vi "DriveHalt.vi"(1 "Parameter String":string, 2 "Reinit":bool) -> (0 "Increment":bool)   [LabVIEW 2019]
uses:
  dsinstructions.vi
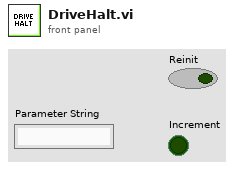
[diagram p1: front panel]
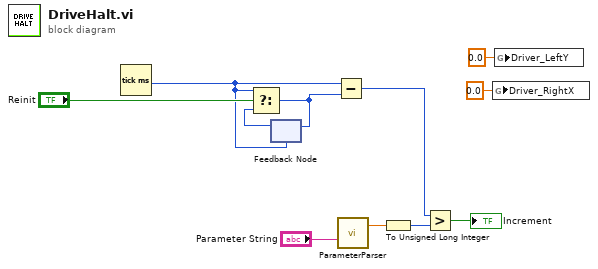
[diagram p0: block diagram]
diagram:
  n1 = Tick Count (ms)() -> (millisecond timer value=w4:u32)
  n2 = feedback #1(w4) -> (w10:u32)
  n3 = Select(t=w4, s="Reinit", f=w10) -> (s? t:f=w8:u32)
  n4 = feedback-in #1(w8) -> ()
  n5 = Subtract(x=w4, y=w8) -> (x-y=w7:u32)
  n6 = call "ParameterParser.vi"("Parameter String"="Parameter String") -> ("Parameter"=w2:dbl)  [unwired: 1 in, 1 out]
  n7 = To Unsigned Long Integer(number=w2) -> (unsigned 32bit integer=w1:u32)
  n8 = Greater?(x=w7, y=w1) -> (0:→"Increment":bool)
  n9 = global write "dsinstructions.vi" "Driver_RightX"(0.0 ("Driver_RightX")) -> ()
  n10 = global write "dsinstructions.vi" "Driver_LeftY"(0.0 ("Driver_LeftY")) -> ()
